vi "SymmetrierungMessdaten.vi"(6 "error in":errorcluster, 7 "Input Array":dbl[](array[numeric])) -> (0 "error out":errorcluster, 1 "xausgleich":dbl format="%#_6f", 2 "Output Array":dbl[](array[numeric]), 3 "xmax":dbl, 4 "xmin":dbl)   [LabVIEW 2016]
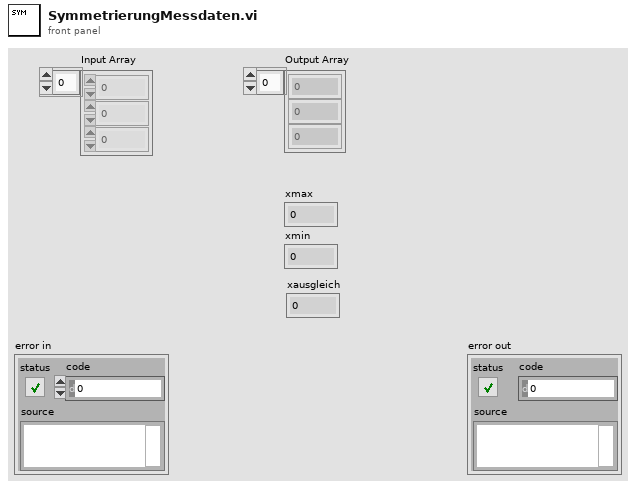
[diagram p1: front panel]
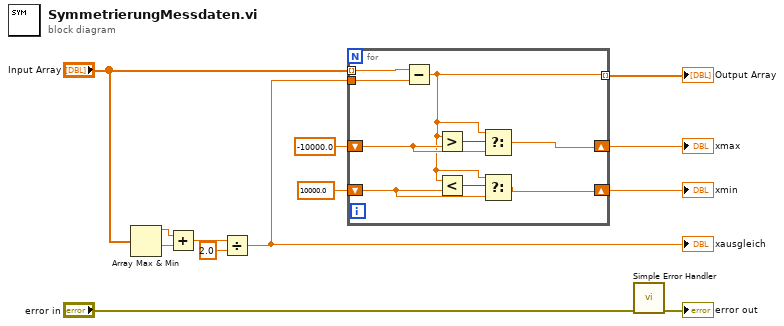
[diagram p0: block diagram]
diagram:
  n1 = Array Max & Min(array="Input Array") -> (max value=w8:dbl, min value=w7:dbl)  [unwired: 2 out]
  n2 = Add(x=w8, y=w7) -> (x+y=w13:dbl)
  n3 = Divide(x=w13, y=2.0) -> (x/y=w10:dbl)
  "xausgleich" <- w10
  n4 = for {
    tunnel: "Input Array" -> [w17] mode=indexing
    tunnel: w10 -> [w22]
    tunnel: [w14] -> w11 mode=indexing
    shift-right: [w19] -> w5
    shift-left: -10000.0 -> [w20]
    shift-right: [w15] -> w4
    shift-left: 10000.0 -> [w16]
    n5 = Subtract(x=w17, y=w22) -> (x-y=w14:dbl)
    n6 = Greater?(x=w14, y=w20) -> (0:w21:bool)
    n7 = Less?(x=w14, y=w16) -> (x < y?=w18:bool)
    n8 = Select(t=w14, s=w21, f=w20) -> (s? t:f=w19:dbl)
    n9 = Select(t=w14, s=w18, f=w16) -> (s? t:f=w15:dbl)
  }
  "Output Array" <- w11
  "xmax" <- w5
  "xmin" <- w4
  n10 = call <vilib>:"Simple Error Handler.vi"("error in (no error)"="error in") -> ("error out"=→"error out":errorcluster)  [unwired: 4 in, 4 out]
